vi "Griddy Score.vi"(11 "Griddy Command":T1) -> ()   [LabVIEW 2020]
uses:
  intake sub/Implementation/Typedef/intake typedef.ctl
  manipulator/Implementation/Typedefs/Teleop Manipulator Commands.ctl
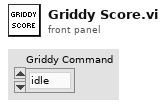
[diagram p1: front panel]
types:
  T1 = typedef "Teleop Manipulator Commands.ctl" = enum16{"idle", "intake cone", "intake cube", "score low cone", "score low cube", "score mid cone", "score mid cube", "score high cone", "score high cube"}
  T2 = typedef "intake typedef.ctl" = enum16{"Intake Cone", "Intake Cube", "Outtake/Score"}
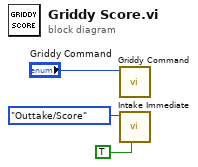
[diagram p0: block diagram]
diagram:
  n1 = call "Griddy Command.vi"("Griddy Command"="Griddy Command") -> ()  [unwired: 10 in, 1 out]
  n2 = call "Intake Immediate.vi"("Wait for Manipulator"=TRUE, "intake modes"=intake_typedef."Outtake/Score") -> ()  [unwired: 9 in, 1 out]
